vi "Edit Configuration.vi"() -> ()   [LabVIEW 2015]
uses:
  Type/_Instrument Model.ctl
  Type/_RT Command.ctl
  Configuration/_Global Configuration.vi
  <vilib>/Utility/config.llb/Read Key (Path).vi
  <vilib>/Utility/config.llb/Read Key (String).vi
  <vilib>/Utility/config.llb/Read Key (I32).vi
  <vilib>/Utility/config.llb/Read Key (Boolean).vi
  <vilib>/Utility/config.llb/Write Key (Path).vi
  <vilib>/Utility/config.llb/Write Key (String).vi
  <vilib>/Utility/config.llb/Write Key (I32).vi
  <vilib>/Utility/config.llb/Write Key (Boolean).vi
  <vilib>/Utility/config.llb/NI_LVConfig.lvlib
panel:
  in  "Update Poles":bool
  in  "Pole Swap Options Negative":T1
  in  "Pole Swap Options Positive":T1
  in  "Enable Voltage Reset":bool=TRUE
  in  "Model Name":T2=enum."IONICS 3Q 220"
  in  "Restore From Power Failure":bool
  out "Num":i32
  in  "Oscillator Settings":string[](array[string])=["", "", ""]
  in  "Settling Time (mS)":dbl=5.0 min=0.0 format="%#.6g"
  in  "User -ve Default":dbl=400.0 format="%#.6g"
  out "# of Parameters":i32=52
  in  "Import":bool
  in  "Export":bool
  in  "S Switch T (mS)":i32=200 min=0
  in  "Pol Switch T (mS)":i32=200 min=0
  in  "CAD Evac T (mS)":i32=5000 min=0
  in  "CAD Fill T (mS)":i32=5000 min=0
  in  "Configuration File Name":string="C:\\Users\\Min\\Projects\\Sniffer\\Build\\Config-090903_virtual_chs.c3n"
  in  "Description":string="Quadrupole 1 RF"
  in  "Type":u8=64 format="%08b"
  in  "Use DT Correction":bool
  in  "Dead Time (nS)":i32=50
  in  "File Path":path=path "C:/Users/Min/Projects/Sniffer/Build/Config-090727_virtual_chs.c3n"
  in  "Reconnect":bool
  in  "IP Address":string="172.16.0.2"
  in  "Serial Number":string="Ionica SN100003A"
  in  "Calibration Offset":dbl format="%#.6g"
  in  "Calibration Slope":dbl=218.45 format="%#.6g"
  in  "User +ve Default":dbl=400.0 format="%#.6g"
  in  "User Maximum":dbl=1600.0 format="%#.6g"
  in  "User Minimum":dbl=15.0 format="%#.6g"
  in  "Channel Number":u8=1 min=1
  in  "Save":bool
  in  "Load":bool
  in  "Undo":bool
  in  "Parameter Name":string="Q1 RF"
  in  "Insert Row":bool
  in  "Delete Row":bool
  in  "Table":i32(listbox)
  # "(Select a current parameter for editing by selecting a row on the table above)"
  # "Current Parameter"
  # "Other Instrument Configurations"
  # "Pole Orientation"
  # "Positive"
  # "Negative"
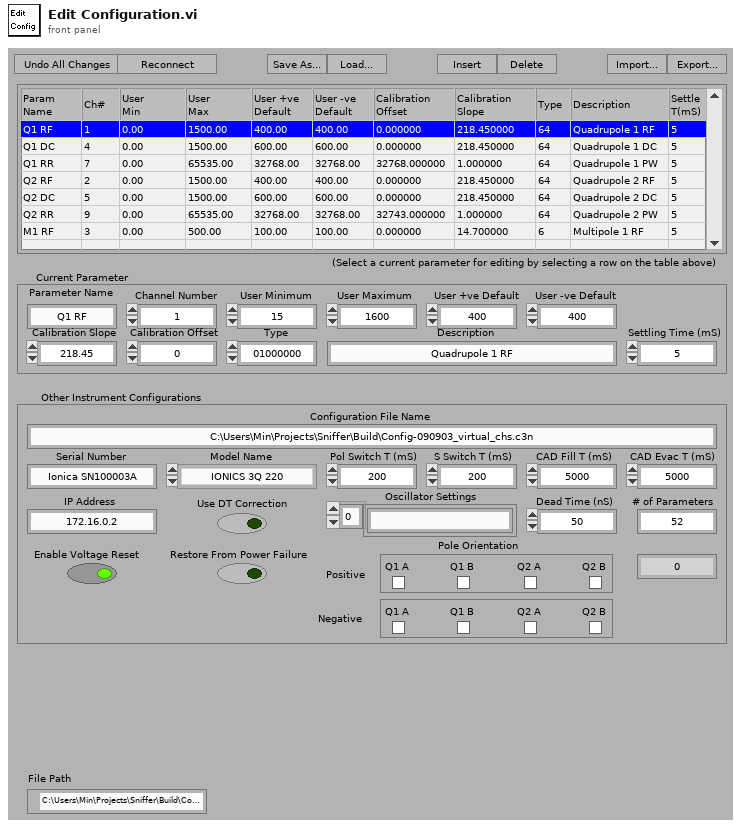
[diagram p1: front panel]
types:
  T1 = cluster{"Q1 A":bool, "Q1 B":bool, "Q2 A":bool, "Q2 B":bool}
  T2 = typedef "_Instrument Model.ctl" = enum16{"QSight 110", "QSight 120", "QSight 210", "QSight 220", "IONICS 3Q 110", "IONICS 3Q 120", "IONICS 3Q 210", "IONICS 3Q 220", "IONICS 3Q 310", "IONICS 3Q 320", "Simulation (Single Source)", "Simulation (Dual Source)"}
  T3 = typedef "_RT Command.ctl" = enum16{"xml Start Run", "xml Start Actual Run", "xml Stop Run", "xml Runtime Update", "xml Get Status", "xml Get Table", "xml Set Table", "xml Get Configuration", "xml System Status", "xml Set LC Input Logic", "xml Get Data", "xml Get Info", "Start", "StartActualRun", "Stop", "Runtime Update", "Get Data", "Get Info", "Get Status", "Get Param", "Get Config", "Get Table", "Read ADC", "Set Oscillator", "Update Config", "Update Table", "Set All Pol", "Set Pol and DC", "Set Max Mass", "Toggle RP", "Toggle EL", "Set PIC", "Initialize Turbo", "Send Turbo Comm", "Close Turbo", "P1", "P2", "P3", "Send Serial", "Set LC Out", "Get LC In", "Read VAC", "Test Table", "Toggle Power", "Get Startup", "Set Startup", "Get ADC Table", "Set ADC Table", "Get Brief Status", "Get Detail Status", "Auxiliary Update", "Set CC Logics", "Set CC Input Logics", "Ignore Error", "invalid"}
  T4 = typedef "NI_LVConfig.lvlib/Config Data RefNum.ctl" = refnum<k1>
  T5 = typedef "_RT Instrument 2.ctl" = cluster{"Table":T6[], "Instrument":string[]}
  T6 = typedef "_RT Configuration 2.ctl" = cluster{"Name":string, "Ch#":u8, "Min":dbl, "Max":dbl, "Def+":dbl, "Def-":dbl, "Offset":dbl, "Slope":dbl, "Type":u8, "Description":string, "SettleT":dbl}
  T7 = cluster{"IP Address":string, "Configuration 2":T5, "Index":i32, "Update Table":bool, "File Path":path}
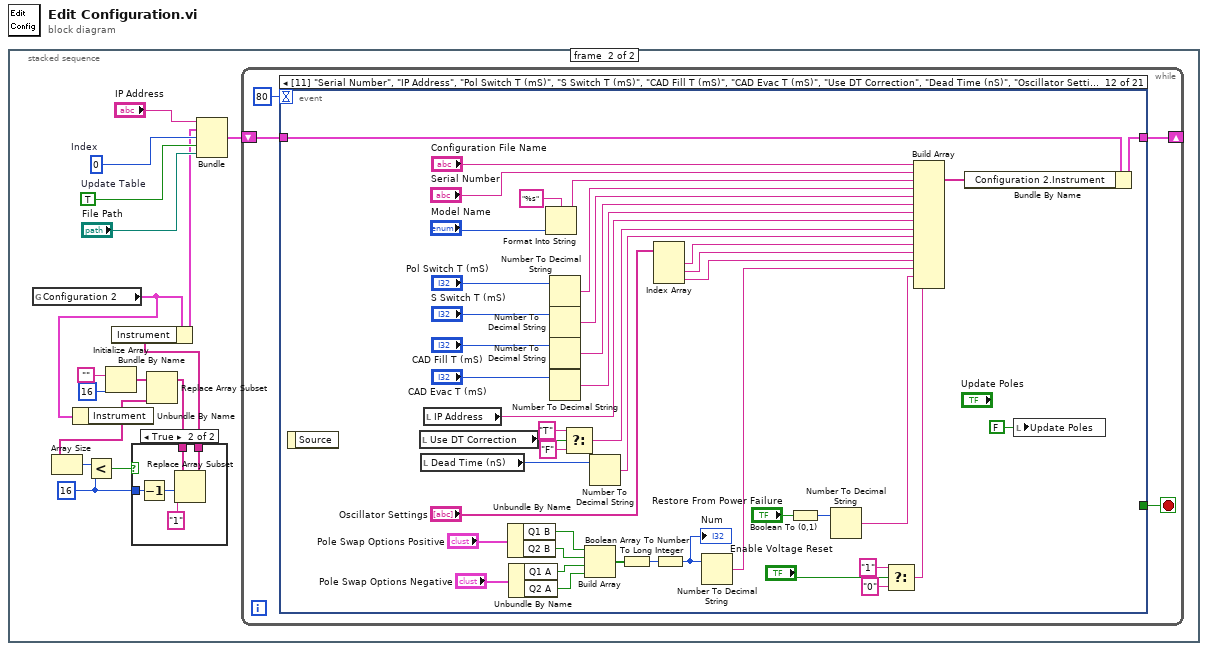
[diagram p0: block diagram]
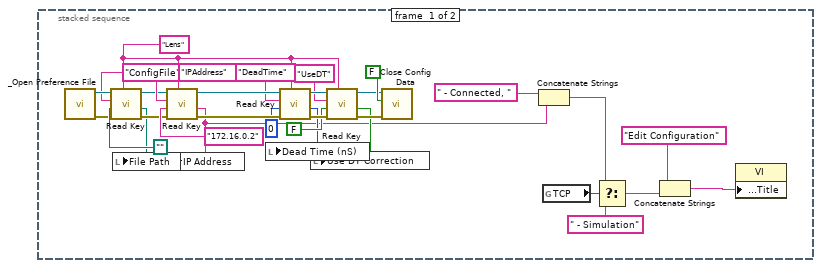
[diagram p2: hidden frame]
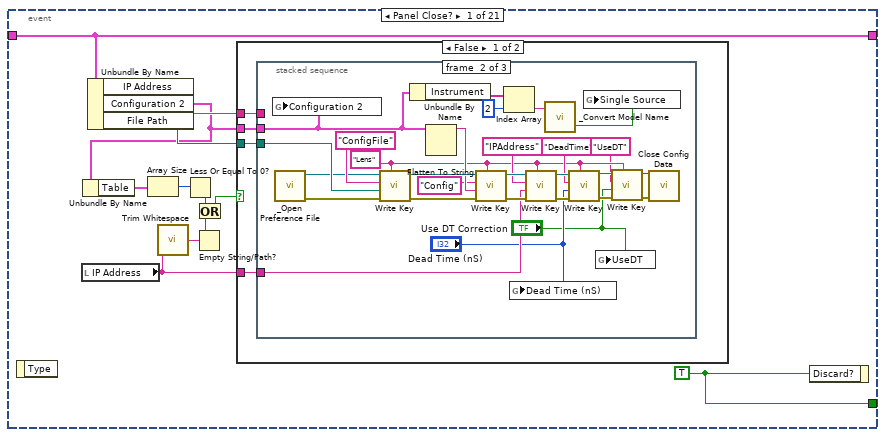
[diagram p4: hidden frame]
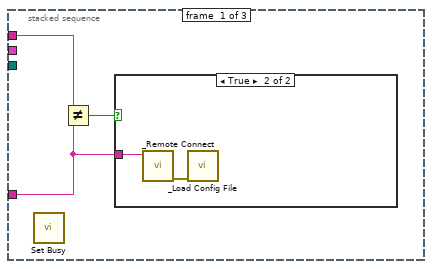
[diagram p5: hidden frame]
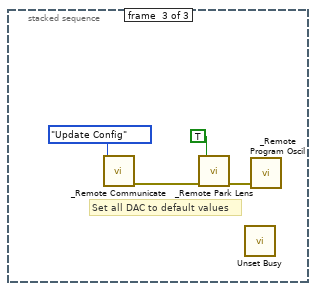
[diagram p7: hidden frame]
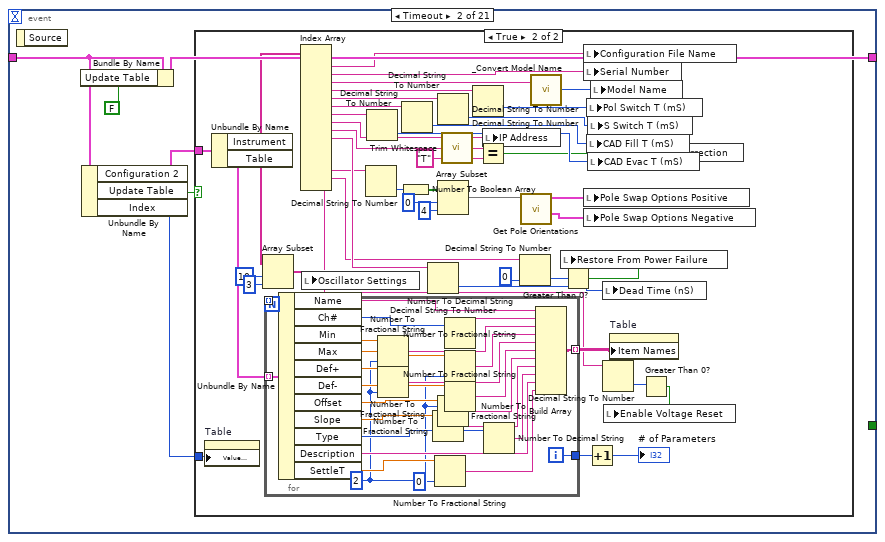
[diagram p9: hidden frame]
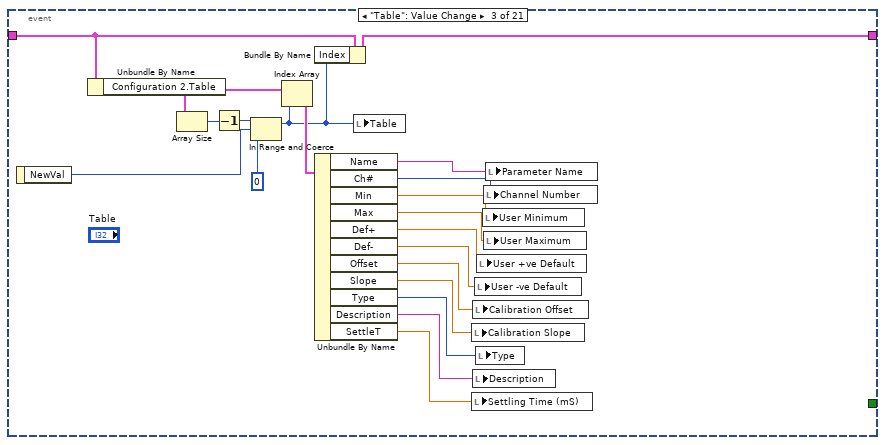
[diagram p11: hidden frame]
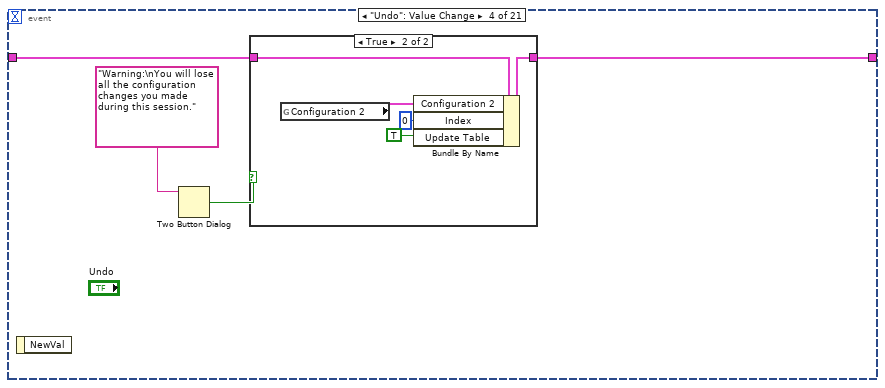
[diagram p12: hidden frame]
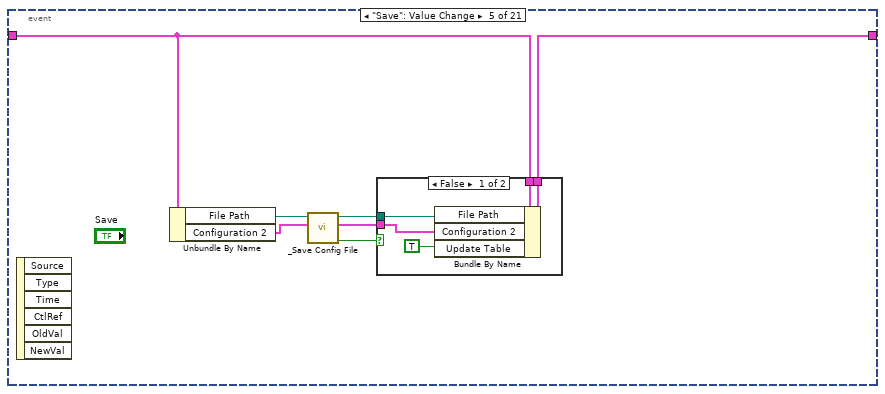
[diagram p14: hidden frame]
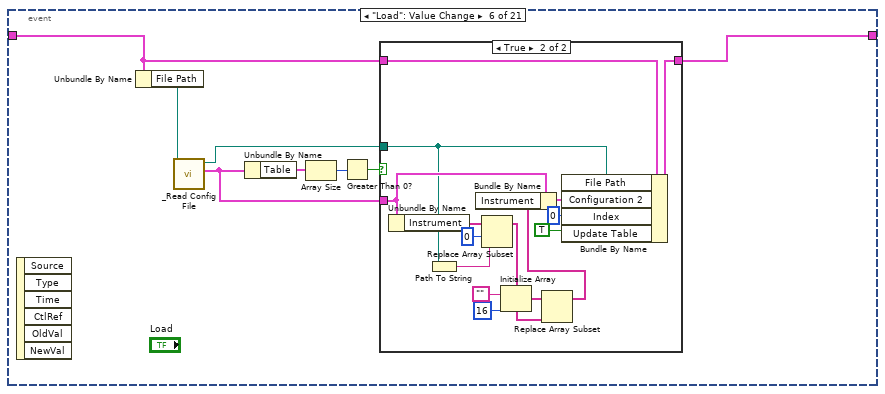
[diagram p16: hidden frame]
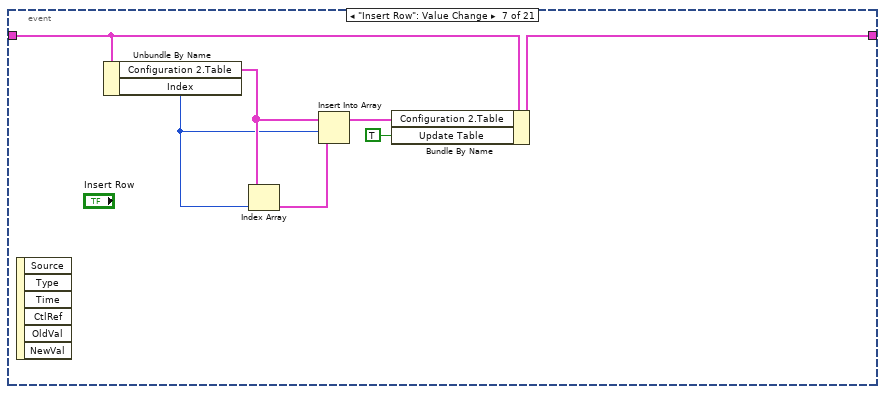
[diagram p18: hidden frame]
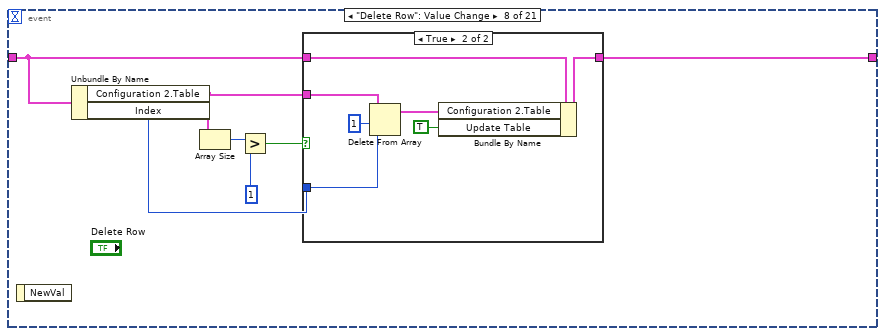
[diagram p19: hidden frame]
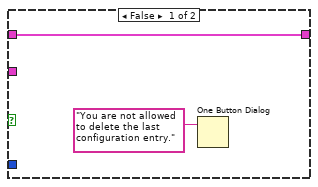
[diagram p20: hidden frame]
diagram:
  n1 = stacked-sequence {
    frame #0 {
      w11 = "Lens" ("section")
      n2 = call "_Open Preference File.vi"() -> ("error"=w24:errorcluster, "refnum"=w23:T4)  [unwired: 3 in, 3 out]
      n3 = call-poly <vilib>:"Read Key.vi"("section"=w11, "error in (no error)"=w24, "default value"=path "", "key"="ConfigFile", "refnum"=w23) -> ("error out"=w27:errorcluster, "value"=w6:path, "refnum out"=w26:T4)  [unwired: 4 out]
      n4 = local write "File Path"(w6) -> ()
      n5 = call-poly <vilib>:"Read Key.vi"("section"=w11, "error in (no error)"=w27, "default value"="172.16.0.2", "key"="IPAddress", "refnum"=w26) -> ("error out"=w19:errorcluster, "value"=w2:string, "refnum out"=w20:T4)  [unwired: 1 in, 3 out]
      n6 = local write "IP Address"(w2) -> ()
      n7 = call-poly <vilib>:"Read Key.vi"("section"=w11, "error in (no error)"=w19, "default value"=0, "key"="DeadTime", "refnum"=w20) -> ("error out"=w16:errorcluster, "value"=w4:i32, "refnum out"=w15:T4)  [unwired: 4 out]
      n8 = local write "Dead Time (nS)"(w4) -> ()
      n9 = call-poly <vilib>:"Read Key.vi"("section"=w11, "error in (no error)"=w16, "default value"=FALSE, "key"="UseDT", "refnum"=w15) -> ("error out"=w12:errorcluster, "value"=w5:bool, "refnum out"=w13:T4)  [unwired: 4 out]
      n10 = local write "Use DT Correction"(w5) -> ()
      n11 = call <vilib>:"Close Config Data.vi"("error in (no error)"=w12, "write file if changed (T)"=FALSE ("write configuration file? (F)"), "refnum"=w13) -> ()  [unwired: 9 out]
      n12 = Concatenate Strings(" - Connected, " ("string"), w2) -> (w1:string)
      n13 = global read "_Global Configuration.vi" "TCP"() -> (w9:bool)
      n14 = Select(t=w1, s=w9, f=" - Simulation" ("string")) -> (s? t:f=w7:string)
      n15 = Concatenate Strings("Edit Configuration" ("string"), w7) -> (w31:string)
      n16 = property class="VI"("Front Panel Window:Title"=w31) -> ()  [unwired: 2 in, 2 out]
    }
    frame #1 {
      w35 = 16 ("dimension size")
      w45 = 0  # Index
      w46 = TRUE  # Update Table
      n17 = global read "_Global Configuration.vi" "Configuration 2"() -> (w42:T5)
      n18 = Unbundle By Name(w42) -> ("Instrument"=w38:string[])
      n19 = Array Size(array=w38) -> (size(s)=w37:i32)
      n20 = Less?(x=w37, y=w35) -> (x < y?=w33:bool)
      n21 = Initialize Array("", 16 ("dimension size")) -> (w39:string[])
      n22 = Replace Array Subset(array=w39, new element=w38) -> (w36:string[])  [unwired: 1 in]
      n23 = case shown="True" w33 {
        tunnel: w36 -> [w48 w53]
        tunnel: w35 -> [_ w52]
        tunnel: [w48 w49] -> w34
        frame False {
        }
        frame True {
          n24 = Decrement(x=w52) -> (x-1=w51:i32)
          n25 = Replace Array Subset(array=w53, new element="1" ("new element/subarray"), index=w51) -> (w49:string[])
        }
      }
      n26 = Bundle By Name(cluster=w42, "Instrument"=w34) -> (w32:T5)
      n27 = Bundle("IP Address"="IP Address", "Configuration 2"=w32, "Index"=w45, "Update Table"=w46, "File Path"="File Path") -> (w47:T7)  [unwired: 1 out]
      n28 = while {
        shift-right: [w55] -> _
        shift-left: w47 -> [w56]
        stop <- w57 stop-if-true
        n29 = event shown="[11] \"Serial Number\", \"IP Address\", \"Pol Switch T (mS)\", \"S Switch T (mS)\", \"CAD Fill T (mS)\", \"CAD Evac T (mS)\", \"Use DT Correction\", \"Dead Time (nS)\", \"Oscillator Settings\", \"Restore From Power Failure\", \"Model Name\", \"Enable Voltage Reset\", \"Update Poles\": Value Change" {
          selector: _ -> [_ _ _ _ _ _ _ _ _ _ _ _ _ _ _ _ _ _ _ _ _]
          dyn-events: _ -> [_ _ _ _ _ _ _ _ _ _ _ _ _ _ _ _ _ _ _ _ _]
          timeout: 80 -> [_ _ _ _ _ _ _ _ _ _ _ _ _ _ _ _ _ _ _ _ _]
          tunnel: [w69 _ _ _ _ _ _ _ _ _ _ _ _ _ _ _ _ _ _ _ _] -> w57
          tunnel: w56 -> [w68 w112 w197 w208 w219 w236 w259 w263 w280 w291 w306 w355 w356 w362 w368 w374 w382 w388 w394 w400 w405]
          tunnel: [w68 w111 w195 w207 w218 w237 w258 w264 w281 w291 w305 w354 w356 w362 w368 w374 w382 w388 w394 w400 w406] -> w55
          event Panel Close? {
            w69 = TRUE ("Discard?")
            n30 = event-data() -> ()  [unwired: 2 out]
            n31 = local read "IP Address"() -> (w62:string)
            n32 = Unbundle By Name(w68) -> ("IP Address"=w67:string, "Configuration 2"=w65:T5, "File Path"=w66:path)
            n33 = Unbundle By Name(w65) -> ("Table"=w64:T6[])
            n34 = Array Size(array=w64) -> (size(s)=w63:i32)
            n35 = call <vilib>:"Trim Whitespace.vi"("string"=w62) -> ("trimmed string"=w61:string)  [unwired: 1 in]
            n36 = Less Or Equal To 0?(x=w63) -> (x <= 0?=w60:bool)
            n37 = Empty String/Path?(string/path=w61) -> (empty?=w59:bool)
            n38 = Or(x=w60, y=w59) -> (x .or. y?=w58:bool)
            n39 = case shown="False" w58 {
              tunnel: w67 -> [w73 _]
              tunnel: w65 -> [w72 _]
              tunnel: w66 -> [w71 _]
              tunnel: w62 -> [w70 _]
              frame False {
                n40 = stacked-sequence {
                  tunnel: w73 -> [w75 _ _]
                  tunnel: w72 -> [_ w81 _]
                  tunnel: w71 -> [_ w105 _]
                  tunnel: w70 -> [w74 w95 _]
                  frame #0 {
                    n41 = call <vilib>:"Set Busy.vi"() -> ()  [unwired: 4 in, 8 out]
                    n42 = Not Equal?(x=w75, y=w74) -> (x != y?=w76:bool)
                    n43 = case shown="True" w76 {
                      tunnel: w74 -> [_ w78]
                      frame False {
                      }
                      frame True {
                        n44 = call "_Remote Connect.vi"("IP Address"=w78) -> ("error out"=w77:errorcluster)  [unwired: 1 in, 5 out]
                        n45 = call "_Load Config File.vi"("error in (no error)"=w77) -> ()  [unwired: 7 out]
                      }
                    }
                  }
                  frame #1 {
                    w86 = "Lens" ("section")
                    n46 = global write "_Global Configuration.vi" "Configuration 2"(w81) -> ()
                    n47 = call "_Open Preference File.vi"() -> ("error"=w98:errorcluster, "refnum"=w99:T4)  [unwired: 3 in, 3 out]
                    n48 = call-poly <vilib>:"Write Key.vi"("section"=w86, "error in (no error)"=w98, "value"=w105, "key"="ConfigFile", "refnum"=w99) -> ("error out"=w97:errorcluster, "refnum out"=w104:T4)  [unwired: 5 out]
                    n49 = Unbundle By Name(w81) -> ("Instrument"=w83:string[])
                    n50 = Flatten To String(anything=w81) -> (data string=w103:string)  [unwired: 1 in, 4 out]
                    n51 = call-poly <vilib>:"Write Key.vi"("section"=w86, "error in (no error)"=w97, "value"=w103, "key"="Config" ("section"), "refnum"=w104) -> ("error out"=w96:errorcluster, "refnum out"=w101:T4)  [unwired: 1 in, 4 out]
                    n52 = Index Array(array=w83, index=2) -> (element=w80:string)
                    n53 = global write "_Global Configuration.vi" "Dead Time (nS)"("Dead Time (nS)") -> ()
                    n54 = call-poly <vilib>:"Write Key.vi"("section"=w86, "error in (no error)"=w96, "value"=w95, "key"="IPAddress" ("section"), "refnum"=w101) -> ("error out"=w94:errorcluster, "refnum out"=w93:T4)  [unwired: 1 in, 4 out]
                    n55 = call "_Convert Model Name.vi"("Model"=w80) -> ("SingleSource"=w79:bool)  [unwired: 1 in, 1 out]
                    n56 = call-poly <vilib>:"Write Key.vi"("section"=w86, "error in (no error)"=w94, "value"="Dead Time (nS)", "key"="DeadTime", "refnum"=w93) -> ("error out"=w90:errorcluster, "refnum out"=w89:T4)  [unwired: 5 out]
                    n57 = global write "_Global Configuration.vi" "Single Source"(w79) -> ()
                    n58 = global write "_Global Configuration.vi" "UseDT"("Use DT Correction") -> ()
                    n59 = call-poly <vilib>:"Write Key.vi"("section"=w86, "error in (no error)"=w90, "value"="Use DT Correction", "key"="UseDT", "refnum"=w89) -> ("error out"=w87:errorcluster, "refnum out"=w88:T4)  [unwired: 5 out]
                    n60 = call <vilib>:"Close Config Data.vi"("error in (no error)"=w87, "refnum"=w88) -> ()  [unwired: 1 in, 9 out]
                  }
                  frame #2 {
                    # "Set all DAC to default values"
                    n61 = call "_Remote Communicate.vi"("Command"=_RT_Command."Update Config") -> ("error out"=w108:errorcluster)  [unwired: 5 in, 3 out]
                    n62 = call "_Remote Park Lens.vi"("error in"=w108, "All Ch (F)"=TRUE) -> ("error out"=w107:errorcluster)  [unwired: 5 out]
                    n63 = call <vilib>:"Unset Busy.vi"() -> ()  [unwired: 2 in, 10 out]
                    n64 = call "_Remote Program Oscil.vi"("error in (no error)"=w107) -> ()  [unwired: 1 out]
                  }
                }
              }
              frame True {
              }
            }
            n65 = event-data("Discard?"=w69) -> ()  [unwired: 1 in, 1 out]
          }
          event Timeout {
            n66 = event-data() -> ()  [unwired: 2 out]
            n67 = Bundle By Name(cluster=w112, "Update Table"=FALSE) -> (w111:T7)
            n68 = Unbundle By Name(w112) -> ("Configuration 2"=w116:T5, "Update Table"=w115:bool, "Index"=w114:i32)
            n69 = case shown="True" w115 {
              tunnel: w116 -> [_ w160]
              tunnel: w114 -> [_ w157]
              frame False {
              }
              frame True {
                n70 = property on="Table" class="MCListbox (strict)"("Value (Signaling)"=w157) -> ()  [unwired: 2 in, 2 out]
                n71 = Unbundle By Name(w160) -> ("Instrument"=w137:string[], "Table"=w159:T6[])
                n72 = Array Subset(array=w137, index=10, length=3) -> (w135:string[])
                n73 = for {
                  N -> [w161]
                  tunnel: w159 -> [w186] mode=indexing
                  tunnel: [w173] -> w158 mode=indexing
                  tunnel: [w169] -> w139
                  tunnel: [w161] -> _ mode=indexing
                  i -> [w169]
                  w163 = i16 2 ("precision (6)")
                  n74 = Unbundle By Name(w186) -> ("Name"=w172:string, "Ch#"=w185:u8, "Min"=w183:dbl, "Max"=w182:dbl, "Def+"=w181:dbl, "Def-"=w180:dbl, "Offset"=w179:dbl, "Slope"=w171:dbl, "Type"=w168:u8, "Description"=w166:string, "SettleT"=w165:dbl)
                  n75 = Number To Fractional String(number=w183, precision (6)=w163) -> (F-format string=w178:string)  [unwired: 2 out]
                  n76 = Number To Fractional String(number=w181, precision (6)=w163) -> (F-format string=w176:string)  [unwired: 2 out]
                  n77 = Number To Fractional String(number=w171) -> (F-format string=w170:string)  [unwired: 3 out]
                  n78 = Number To Fractional String(number=w165, precision (6)=i16 0) -> (F-format string=w164:string)  [unwired: 2 out]
                  n79 = Number To Fractional String(number=w179) -> (F-format string=w174:string)  [unwired: 3 out]
                  n80 = Number To Decimal String(number=w185) -> (decimal integer string=w184:string)  [unwired: 1 out]
                  n81 = Number To Fractional String(number=w182, precision (6)=w163) -> (F-format string=w177:string)  [unwired: 2 out]
                  n82 = Number To Fractional String(number=w180, precision (6)=w163) -> (F-format string=w175:string)  [unwired: 2 out]
                  n83 = Number To Decimal String(number=w168) -> (decimal integer string=w167:string)  [unwired: 1 out]
                  n84 = Build Array(w172, w184, w178, w177, w176, w175, w174, w170, w167, w166, w164) -> (w173:string[])
                }
                n85 = Index Array(array=w137) -> (element #1=w156:string, element #2=w155:string, element #3=w124:string, element #4=w154:string, element #5=w153:string, element #6=w151:string, element #7=w150:string, element #8=w146:string, element #9=w143:string, element #10=w144:string, element #14=w126:string, element #15=w133:string, element #16=w120:string)  [unwired: 16 in, 3 out]
                n86 = local write "Oscillator Settings"(w135) -> ()
                n87 = Decimal String To Number(string=w126) -> (number=w127:i32)  [unwired: 3 out]
                n88 = Decimal String To Number(string=w150) -> (number=w147:i32)  [unwired: 3 out]
                n89 = Number To Boolean Array(number=w127) -> (Boolean array=w128:bool[])
                n90 = Decimal String To Number(string=w151) -> (number=w148:i32)  [unwired: 3 out]
                n91 = Decimal String To Number(string=w144) -> (number=w145:i32)  [unwired: 3 out]
                n92 = Decimal String To Number(string=w153) -> (number=w149:i32)  [unwired: 3 out]
                n93 = Array Subset(array=w128, index=0, length=4) -> (w119:bool[])
                n94 = call <vilib>:"Trim Whitespace.vi"("string"=w143) -> ("trimmed string"=w142:string)  [unwired: 1 in]
                n95 = Decimal String To Number(string=w154) -> (number=w152:i32)  [unwired: 3 out]
                n96 = Equal?(x=w142, y="T") -> (x = y?=w140:bool)
                n97 = local write "IP Address"(w146) -> ()
                n98 = Decimal String To Number(string=w133, default (0L)=0 ("default (0 I32)")) -> (number=w132:i32)  [unwired: 2 out]
                n99 = call "Get Pole Orientations.vi"("Pole"=w119) -> ("Pole Swap Options Negative"=w117:T1, "Pole Swap Options Positive"=w118:T1)  [unwired: 9 in]
                n100 = call "_Convert Model Name.vi"("Model"=w124) -> ("Model Name"=w123:T2)  [unwired: 1 in, 1 out]
                n101 = Greater Than 0?(x=w132) -> (x > 0?=w125:bool)
                n102 = local write "Restore From Power Failure"(w125) -> ()
                n103 = local write "Configuration File Name"(w156) -> ()
                n104 = local write "Serial Number"(w155) -> ()
                n105 = local write "Pole Swap Options Positive"(w118) -> ()
                n106 = local write "Pole Swap Options Negative"(w117) -> ()
                n107 = local write "Pol Switch T (mS)"(w152) -> ()
                n108 = local write "CAD Fill T (mS)"(w148) -> ()
                n109 = Increment(x=w139) -> (x+1=→"# of Parameters":i32)
                n110 = local write "S Switch T (mS)"(w149) -> ()
                n111 = local write "CAD Evac T (mS)"(w147) -> ()
                n112 = local write "Model Name"(w123) -> ()
                n113 = local write "Dead Time (nS)"(w145) -> ()
                n114 = Decimal String To Number(string=w120) -> (number=w122:i32)  [unwired: 3 out]
                n115 = property on="Table" class="MCListbox (strict)"("Item Names"=w158) -> ()  [unwired: 2 in, 2 out]
                n116 = local write "Use DT Correction"(w140) -> ()
                n117 = Greater Than 0?(x=w122) -> (x > 0?=w121:bool)
                n118 = local write "Enable Voltage Reset"(w121) -> ()
              }
            }
          }
          event "Table": Value Change {
            n119 = event-data() -> ("NewVal"=w200:i32)  [unwired: 1 out]
            n120 = Unbundle By Name(w197) -> ("Configuration 2.Table"=w199:T6[])
            n121 = Array Size(array=w199) -> (size(s)=w203:i32)
            n122 = Decrement(x=w203) -> (x-1=w201:i32)
            n123 = In Range and Coerce(upper limit=w201, x=w200, lower limit=0) -> (coerced(x)=w196:i32)  [unwired: 1 out]
            n124 = Index Array(array=w199, index=w196) -> (element=w206:T6)
            n125 = Bundle By Name(cluster=w197, "Index"=w196) -> (w195:T7)
            n126 = Unbundle By Name(w206) -> ("Name"=w205:string, "Ch#"=w198:u8, "Min"=w194:dbl, "Max"=w193:dbl, "Def+"=w204:dbl, "Def-"=w188:dbl, "Offset"=w192:dbl, "Slope"=w191:dbl, "Type"=w190:u8, "Description"=w189:string, "SettleT"=w187:dbl)
            n127 = local write "Table"(w196) -> ()
            n128 = local write "Calibration Slope"(w191) -> ()
            n129 = local write "Settling Time (mS)"(w187) -> ()
            n130 = local write "Calibration Offset"(w192) -> ()
            n131 = local write "Description"(w189) -> ()
            n132 = local write "User -ve Default"(w188) -> ()
            n133 = local write "Type"(w190) -> ()
            n134 = local write "User +ve Default"(w204) -> ()
            n135 = local write "User Minimum"(w194) -> ()
            n136 = local write "Channel Number"(w198) -> ()
            n137 = local write "User Maximum"(w193) -> ()
            n138 = local write "Parameter Name"(w205) -> ()
          }
          event "Undo": Value Change {
            n139 = event-data() -> ()  [unwired: 2 out]
            n140 = Two Button Dialog(message="Warning:\nYou will lose all the configuration changes you made during this session.") -> (T button?=w209:bool)  [unwired: 2 out]
            n141 = case shown="True" w209 {
              tunnel: w208 -> [w211 w216]
              tunnel: [w211 w213] -> w207
              frame False {
              }
              frame True {
                n142 = global read "_Global Configuration.vi" "Configuration 2"() -> (w212:T5)
                n143 = Bundle By Name(cluster=w216, "Configuration 2"=w212, "Index"=0 ("Method Index"), "Update Table"=TRUE) -> (w213:T7)
              }
            }
          }
          event "Save": Value Change {
            n144 = event-data() -> ()  [unwired: 7 out]
            n145 = Unbundle By Name(w219) -> ("File Path"=w223:path, "Configuration 2"=w222:T5)
            n146 = call "_Save Config File.vi"("Configuration"=w222, "start path  (Not A Path)"=w223) -> ("error"=w221:bool, "Config Out"=w217:T5, "new file path"=w220:path)  [unwired: 6 in, 1 out]
            n147 = case shown="False" w221 {
              tunnel: w220 -> [w225 _]
              tunnel: w219 -> [w228 w229]
              tunnel: [w227 w229] -> w218
              tunnel: w217 -> [w224 _]
              frame False {
                n148 = Bundle By Name(cluster=w228, "File Path"=w225, "Configuration 2"=w224, "Update Table"=TRUE) -> (w227:T7)
              }
              frame True {
              }
            }
          }
          event "Load": Value Change {
            n149 = event-data() -> ()  [unwired: 7 out]
            n150 = Unbundle By Name(w236) -> ("File Path"=w235:path)
            n151 = call "_Read Config File.vi"("start path  (Not A Path)"=w235) -> ("Configuration"=w230:T5, "new file path"=w234:path)  [unwired: 2 in, 7 out]
            n152 = Unbundle By Name(w230) -> ("Table"=w231:T6[])
            n153 = Array Size(array=w231) -> (size(s)=w233:i32)
            n154 = Greater Than 0?(x=w233) -> (x > 0?=w232:bool)
            n155 = case shown="True" w232 {
              tunnel: w236 -> [w238 w251]
              tunnel: [w238 w250] -> w237
              tunnel: w234 -> [_ w246]
              tunnel: w230 -> [_ w247]
              frame False {
              }
              frame True {
                n156 = Unbundle By Name(w247) -> ("Instrument"=w249:string[])
                n157 = Path To String(path=w246) -> (string=w244:string)
                n158 = Replace Array Subset(array=w249, new element=w244, index=0) -> (w240:string[])
                n159 = Initialize Array("", 16 ("dimension size")) -> (w243:string[])
                n160 = Replace Array Subset(array=w243, new element=w240) -> (w239:string[])  [unwired: 1 in]
                n161 = Bundle By Name(cluster=w247, "Instrument"=w239) -> (w245:T5)
                n162 = Bundle By Name(cluster=w251, "File Path"=w246, "Configuration 2"=w245, "Index"=0 ("Method Index"), "Update Table"=TRUE) -> (w250:T7)
              }
            }
          }
          event "Insert Row": Value Change {
            n163 = event-data() -> ()  [unwired: 7 out]
            n164 = Unbundle By Name(w259) -> ("Configuration 2.Table"=w256:T6[], "Index"=w254:i32)
            n165 = Index Array(array=w256, index=w254) -> (element=w255:T6)
            n166 = Insert Into Array(array=w256, index=w254, new element=w255) -> (w257:T6[])
            n167 = Bundle By Name(cluster=w259, "Configuration 2.Table"=w257, "Update Table"=TRUE) -> (w258:T7)
          }
          event "Delete Row": Value Change {
            n168 = event-data() -> ()  [unwired: 2 out]
            n169 = Unbundle By Name(w263) -> ("Configuration 2.Table"=w262:T6[], "Index"=w261:i32)
            n170 = Array Size(array=w262) -> (size(s)=w267:i32)
            n171 = Greater?(x=w267, y=1) -> (0:w265:bool)
            n172 = case shown="True" w265 {
              tunnel: w263 -> [w268 w271]
              tunnel: [w268 w270] -> w264
              tunnel: w262 -> [_ w276]
              tunnel: w261 -> [_ w275]
              frame False {
                n173 = One Button Dialog(message="You are not allowed to delete the last configuration entry.") -> ()  [unwired: 2 out]
              }
              frame True {
                n174 = Delete From Array(array=w276, length=1, index=w275) -> (array with subset deleted=w272:T6[])  [unwired: 1 out]
                n175 = Bundle By Name(cluster=w271, "Configuration 2.Table"=w272, "Update Table"=TRUE) -> (w270:T7)
              }
            }
          }
          event "Import": Value Change {
            n176 = event-data() -> ()  [unwired: 2 out]
            n177 = Unbundle By Name(w280) -> ("File Path"=w279:path)
            n178 = call "_Read Spreadsheet.vi"("Start Path"=w279) -> ("Table"=w277:T6[], "Succeded"=w278:bool)  [unwired: 2 out]
            n179 = case shown="True" w278 {
              tunnel: w280 -> [w282 w285]
              tunnel: [w282 w284] -> w281
              tunnel: w277 -> [_ w283]
              frame False {
              }
              frame True {
                n180 = Bundle By Name(cluster=w285, "Configuration 2.Table"=w283, "Update Table"=TRUE) -> (w284:T7)
              }
            }
          }
          event "Export": Value Change {
            n181 = event-data() -> ()  [unwired: 2 out]
            n182 = Unbundle By Name(w291) -> ("File Path"=w290:path)
            n183 = property on="Table" class="MCListbox (strict)"() -> ("ColHdrString"=w289:string[], "Item Names"=w288:string[][])  [unwired: 2 in, 2 out]
            n184 = call "_Write Spreadsheet.vi"("Table"=w288, "Titles"=w289, "Start Path"=w290) -> ("error out"=w287:errorcluster)
            n185 = call "_Handle Error.vi"("error in (no error)"=w287) -> ()  [unwired: 2 in, 5 out]
          }
          event "Parameter Name", "Channel Number", "User Minimum", "User Maximum", "User +ve Default", "Calibration Slope", "Calibration Offset", "Type", "Description", "User -ve Default", "Settling Time (mS)": Value Change {
            n186 = event-data() -> ()  [unwired: 2 out]
            n187 = Unbundle By Name(w306) -> ("Configuration 2.Table"=w304:T6[], "Index"=w303:i32)
            n188 = Index Array(array=w304, index=w303) -> (element=w302:T6)
            n189 = Bundle By Name(cluster=w302, "Name"="Parameter Name", "Ch#"="Channel Number", "Min"="User Minimum", "Max"="User Maximum", "Def+"="User +ve Default", "Def-"="User -ve Default", "Offset"="Calibration Offset", "Slope"="Calibration Slope", "Type"="Type", "Description"="Description", "SettleT"="Settling Time (mS)") -> (w310:T6)
            n190 = Replace Array Subset(array=w304, new element=w310, index=w303) -> (w307:T6[])
            n191 = Bundle By Name(cluster=w306, "Configuration 2.Table"=w307, "Update Table"=TRUE) -> (w305:T7)
          }
          event "Serial Number", "IP Address", "Pol Switch T (mS)", "S Switch T (mS)", "CAD Fill T (mS)", "CAD Evac T (mS)", "Use DT Correction", "Dead Time (nS)", "Oscillator Settings", "Restore From Power Failure", "Enable Voltage Reset", "Update Poles": Value Change {
            n192 = event-data() -> ()  [unwired: 2 out]
            n193 = local read "Use DT Correction"() -> (w348:bool)
            n194 = local read "Dead Time (nS)"() -> (w349:i32)
            n195 = local read "IP Address"() -> (w339:string)
            n196 = Unbundle By Name("Pole Swap Options Positive") -> ("Q1 B"=w318:bool, "Q2 B"=w317:bool)
            n197 = Unbundle By Name("Pole Swap Options Negative") -> ("Q1 A"=w316:bool, "Q2 A"=w315:bool)
            n198 = Format Into String(format string="%s", "Model Name") -> (resulting string=w323:string)  [unwired: 2 in, 1 out]
            n199 = Number To Decimal String(number="Pol Switch T (mS)") -> (decimal integer string=w343:string)  [unwired: 1 out]
            n200 = Number To Decimal String(number="S Switch T (mS)") -> (decimal integer string=w342:string)  [unwired: 1 out]
            n201 = Number To Decimal String(number="CAD Fill T (mS)") -> (decimal integer string=w341:string)  [unwired: 1 out]
            n202 = Number To Decimal String(number="CAD Evac T (mS)") -> (decimal integer string=w340:string)  [unwired: 1 out]
            n203 = Select(t="T", s=w348, f="F") -> (s? t:f=w338:string)
            n204 = Build Array(w318, w317, w316, w315) -> (w314:bool[])
            n205 = Number To Decimal String(number=w349) -> (decimal integer string=w337:string)  [unwired: 1 out]
            n206 = Boolean Array To Number(Boolean array=w314) -> (number=w330:u32)
            n207 = Index Array(array="Oscillator Settings") -> (element #1=w334:string, element #2=w333:string, element #3=w332:string)  [unwired: 3 in]
            n208 = To Long Integer(number=w330) -> (32bit integer=w328:i32)
            "Num" <- w328
            n209 = Number To Decimal String(number=w328) -> (decimal integer string=w329:string)  [unwired: 1 out]
            n210 = Boolean To (0,1)(Boolean="Restore From Power Failure") -> (0, 1=w326:i16)
            n211 = Number To Decimal String(number=w326) -> (decimal integer string=w331:string)  [unwired: 1 out]
            n212 = Select(t="1", s="Enable Voltage Reset", f="0") -> (s? t:f=w319:string)
            n213 = Build Array("Configuration File Name", "Serial Number", w323, w343, w342, w341, w340, w339, w338, w337, w334, w333, w332, w329, w331, w319) -> (w336:string[])
            n214 = Bundle By Name(cluster=w355, "Configuration 2.Instrument"=w336) -> (w354:T7)
            n215 = local write "Update Poles"(FALSE ("Update Poles")) -> ()
          }
          event "Pole Swap Options Positive.Q1 A": Value Change {
            n216 = event-data() -> ("NewVal"=w359:bool)  [unwired: 1 out]
            n217 = local read "Pole Swap Options Positive"() -> (w357:T1)
            n218 = Not(x=w359) -> (.not. x?=w361:bool)
            n219 = property on="Update Poles" class="Bool (strict)"("Val(Sgnl)"=TRUE ("Value (Signaling)")) -> ()  [unwired: 2 in, 2 out]
            n220 = Bundle By Name(cluster=w357, "Q1 A"=w359, "Q1 B"=w361) -> (w358:T1)
            n221 = local write "Pole Swap Options Positive"(w358) -> ()
          }
          event "Pole Swap Options Positive.Q1 B": Value Change {
            n222 = event-data() -> ("NewVal"=w365:bool)  [unwired: 1 out]
            n223 = local read "Pole Swap Options Positive"() -> (w363:T1)
            n224 = Not(x=w365) -> (.not. x?=w367:bool)
            n225 = property on="Update Poles" class="Bool (strict)"("Val(Sgnl)"=TRUE ("Value (Signaling)")) -> ()  [unwired: 2 in, 2 out]
            n226 = Bundle By Name(cluster=w363, "Q1 B"=w365, "Q1 A"=w367) -> (w364:T1)
            n227 = local write "Pole Swap Options Positive"(w364) -> ()
          }
          event "Pole Swap Options Positive.Q2 A": Value Change {
            n228 = event-data() -> ("NewVal"=w371:bool)  [unwired: 1 out]
            n229 = local read "Pole Swap Options Positive"() -> (w369:T1)
            n230 = Not(x=w371) -> (.not. x?=w373:bool)
            n231 = property on="Update Poles" class="Bool (strict)"("Val(Sgnl)"=TRUE ("Value (Signaling)")) -> ()  [unwired: 2 in, 2 out]
            n232 = Bundle By Name(cluster=w369, "Q2 A"=w371, "Q2 B"=w373) -> (w370:T1)
            n233 = local write "Pole Swap Options Positive"(w370) -> ()
          }
          event "Pole Swap Options Positive.Q2 B": Value Change {
            n234 = event-data() -> ("NewVal"=w377:bool)  [unwired: 1 out]
            n235 = local read "Pole Swap Options Positive"() -> (w375:T1)
            n236 = Not(x=w377) -> (.not. x?=w379:bool)
            n237 = property on="Update Poles" class="Bool (strict)"("Val(Sgnl)"=TRUE ("Value (Signaling)")) -> ()  [unwired: 2 in, 2 out]
            n238 = Bundle By Name(cluster=w375, "Q2 B"=w377, "Q2 A"=w379) -> (w376:T1)
            n239 = local write "Pole Swap Options Positive"(w376) -> ()
          }
          event "Pole Swap Options Negative.Q1 A": Value Change {
            n240 = event-data() -> ("NewVal"=w383:bool)  [unwired: 1 out]
            n241 = local read "Pole Swap Options Negative"() -> (w381:T1)
            n242 = Not(x=w383) -> (.not. x?=w385:bool)
            n243 = property on="Update Poles" class="Bool (strict)"("Val(Sgnl)"=TRUE ("Value (Signaling)")) -> ()  [unwired: 2 in, 2 out]
            n244 = Bundle By Name(cluster=w381, "Q1 A"=w383, "Q1 B"=w385) -> (w380:T1)
            n245 = local write "Pole Swap Options Negative"(w380) -> ()
          }
          event "Pole Swap Options Negative.Q1 B": Value Change {
            n246 = event-data() -> ("NewVal"=w389:bool)  [unwired: 1 out]
            n247 = local read "Pole Swap Options Negative"() -> (w387:T1)
            n248 = Not(x=w389) -> (.not. x?=w391:bool)
            n249 = property on="Update Poles" class="Bool (strict)"("Val(Sgnl)"=TRUE ("Value (Signaling)")) -> ()  [unwired: 2 in, 2 out]
            n250 = Bundle By Name(cluster=w387, "Q1 B"=w389, "Q1 A"=w391) -> (w386:T1)
            n251 = local write "Pole Swap Options Negative"(w386) -> ()
          }
          event "Pole Swap Options Negative.Q2 A": Value Change {
            n252 = event-data() -> ("NewVal"=w395:bool)  [unwired: 1 out]
            n253 = local read "Pole Swap Options Negative"() -> (w393:T1)
            n254 = Not(x=w395) -> (.not. x?=w397:bool)
            n255 = property on="Update Poles" class="Bool (strict)"("Val(Sgnl)"=TRUE ("Value (Signaling)")) -> ()  [unwired: 2 in, 2 out]
            n256 = Bundle By Name(cluster=w393, "Q2 A"=w395, "Q2 B"=w397) -> (w392:T1)
            n257 = local write "Pole Swap Options Negative"(w392) -> ()
          }
          event "Pole Swap Options Negative.Q2 B": Value Change {
            n258 = event-data() -> ("NewVal"=w401:bool)  [unwired: 1 out]
            n259 = local read "Pole Swap Options Negative"() -> (w399:T1)
            n260 = Not(x=w401) -> (.not. x?=w403:bool)
            n261 = property on="Update Poles" class="Bool (strict)"("Val(Sgnl)"=TRUE ("Value (Signaling)")) -> ()  [unwired: 2 in, 2 out]
            n262 = Bundle By Name(cluster=w399, "Q2 B"=w401, "Q2 A"=w403) -> (w398:T1)
            n263 = local write "Pole Swap Options Negative"(w398) -> ()
          }
          event "Reconnect": Value Change {
            n264 = event-data() -> ()  [unwired: 7 out]
            n265 = flat-sequence {
              tunnel: [w408] -> w407
              tunnel: [w411] -> w404
              tunnel: w407 -> [w421]
              frame #0 {
                n266 = call <vilib>:"Set Busy.vi"() -> ()  [unwired: 4 in, 8 out]
              }
              frame #1 {
                n267 = local read "IP Address"() -> (w411:string)
                n268 = call "_Remote Connect.vi"("IP Address"=w411) -> ("error out"=w409:errorcluster, "TCP"=w410:bool)  [unwired: 1 in, 4 out]
                n269 = case shown="True" w410 {
                  tunnel: "Edit Configuration" ("string") -> [w416 w419]
                  tunnel: [w414 w420] -> w413
                  tunnel: w411 -> [_ w418]
                  frame False {
                    n270 = Concatenate Strings(w416, " - Simulation" ("string")) -> (w414:string)
                  }
                  frame True {
                    n271 = Concatenate Strings(w419, " - Connected, " ("string"), w418) -> (w420:string)
                  }
                }
                n272 = call "_Load Config File.vi"("error in (no error)"=w409) -> ("error out"=w408:errorcluster)  [unwired: 6 out]
                n273 = property class="VI"("Front Panel Window:Title"=w413) -> ()  [unwired: 2 in, 2 out]
              }
              frame #2 {
                n274 = call <vilib>:"Unset Busy.vi"() -> ()  [unwired: 2 in, 10 out]
                n275 = call "_Handle Error.vi"("error in (no error)"=w421) -> ()  [unwired: 2 in, 5 out]
              }
            }
            n276 = Bundle By Name(cluster=w405, "IP Address"=w404) -> (w406:T7)
          }
        }
      }
    }
  }
